vi "color split.vi"(4 "point style":enum16{"dot", "cross"}(ring), 5 "mapping":T1(ring), 6 "tfolder":T3={"tfolder path"=path "/snowfall/Users/arcadi/Desktop/Ultrasound/Experiment/YBCO_4/Round1/Sweep12/June_2011/062511/221.16400K_300_3100_001_062511.dat", "9folder path"=path "/snowfall/Users/arcadi/Desktop/Ultrasound/Experiment/YBCO_4/Round1/Sweep12/June_2011/062511/221.16400K_300_3100_001_062511.dat", "tfolder  -  file array"=[], "from index array"=[], "timestamp array"=[]}, 7 "Plot Ref":refnum<vi>, 8 "plot array IN":T2(array[cluster]), 10 "Y":dbl[](array[numeric]), 11 "X":dbl[](array[numeric])) -> (0 "plot array OUT":T2(array[cluster]))   [LabVIEW 2015]
uses:
  tfolder.ctl
  tfolder -- monotonic segment.ctl
panel:
  in  "output cluster":T5
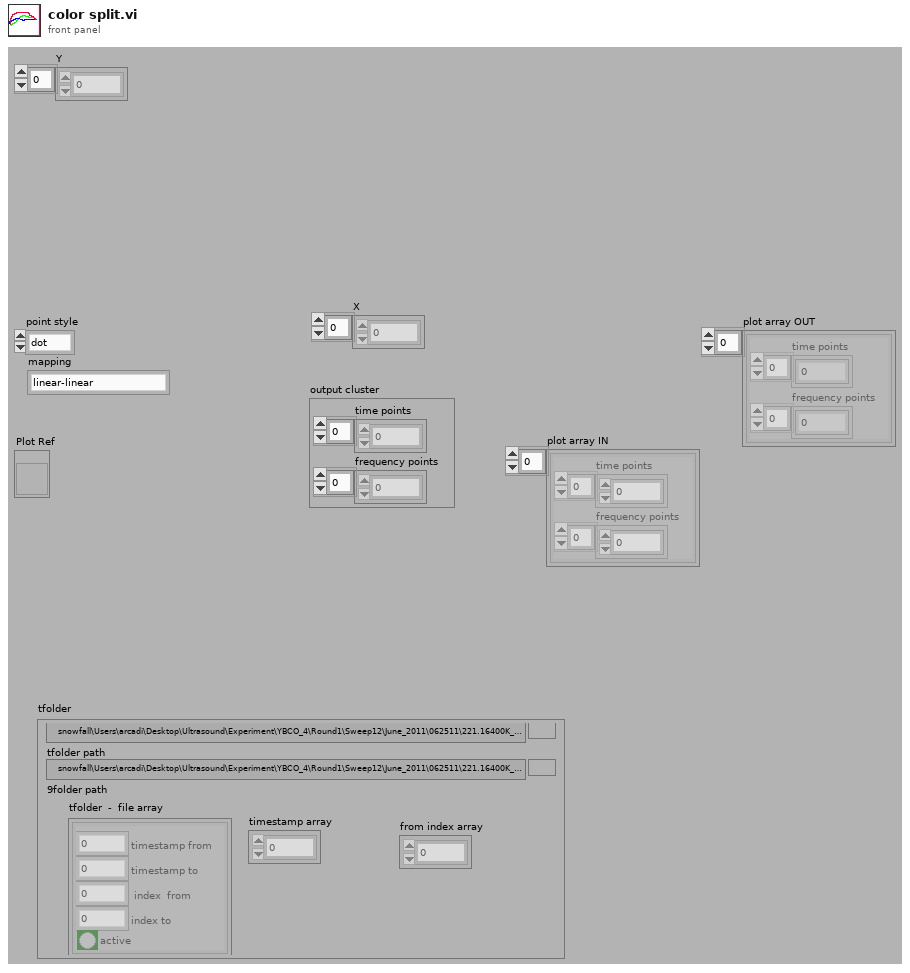
[diagram p1: front panel]
types:
  T1 = enum16{"linear-linear", "log-linear", "linear-log", "log-log"}
  T2 = cluster{"time points":dbl[], "frequency points":dbl[]}[]
  T3 = typedef "tfolder.ctl" = cluster{"tfolder path":path, "9folder path":path, "tfolder  -  file array":T4[], "from index array":i32[], "timestamp array":dbl[]}
  T4 = typedef "tfolder -- monotonic segment.ctl" = cluster{"timestamp from":dbl, "timestamp to":dbl, " index  from":i32, "index to":i32, "active":bool}
  T5 = cluster{"time points":dbl[], "frequency points":dbl[]}
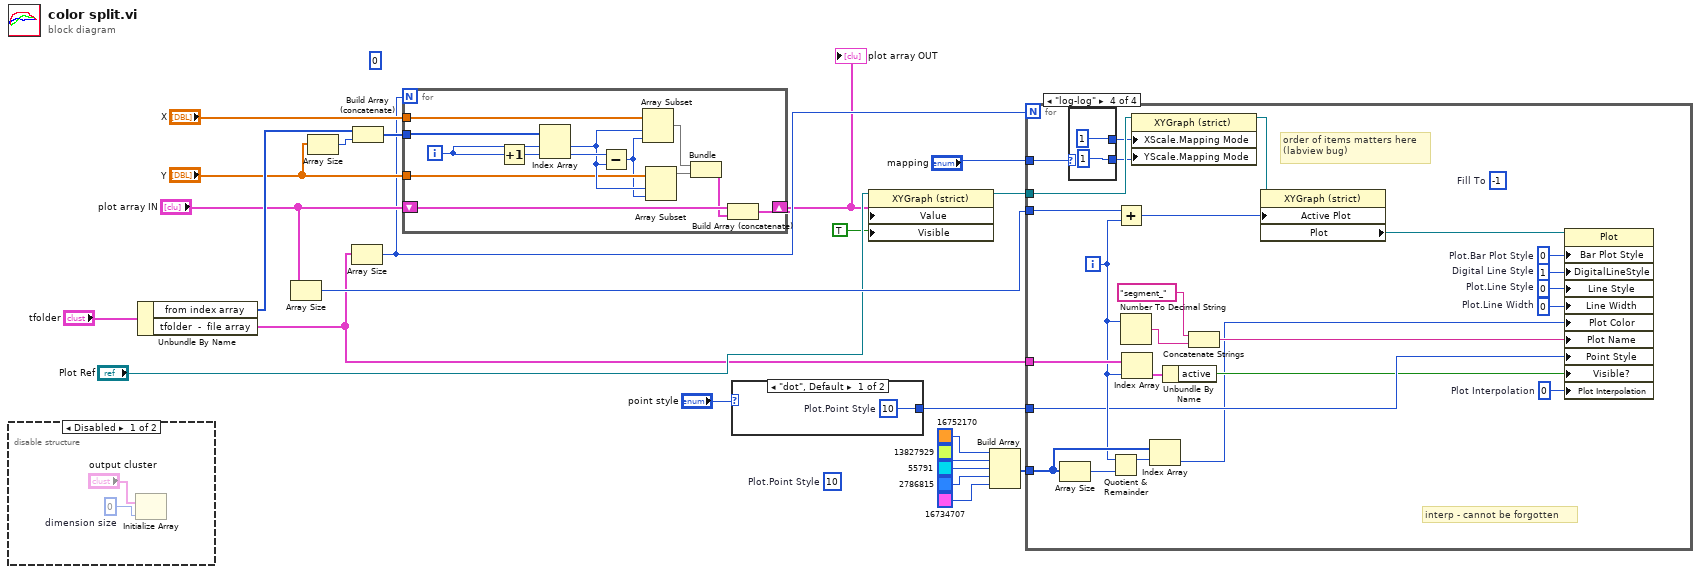
[diagram p0: block diagram]
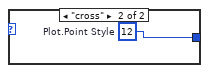
[diagram p2: hidden frame]
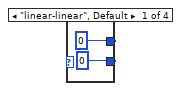
[diagram p4: hidden frame]
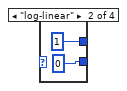
[diagram p5: hidden frame]
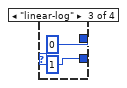
[diagram p6: hidden frame]
diagram:
  (unwired) u8 10  # Plot.Point Style
  (unwired) 0 ("dimension size")
  n1 = disable-structure shown="Disabled" {
    frame Disabled {
      w25 = 0  # dimension size
      n2 = Initialize Array("output cluster", w25) -> ()  [unwired: 1 out]
    }
    frame Enabled {
    }
  }
  n3 = Unbundle By Name("tfolder") -> ("from index array"=w21:i32[], "tfolder  -  file array"=w6:T4[])
  n4 = Array Size(array="plot array IN") -> (size(s)=w16:i32)
  n5 = Array Size(array="Y") -> (size(s)=w22:i32)
  n6 = Array Size(array=w6) -> (size(s)=w9:i32)
  n7 = Build Array (concatenate)(w21, w22) -> (w20:i32[])
  n8 = for {
    N: w9 -> [_]
    shift-right: [w31] -> w7
    shift-left: "plot array IN" -> [w32]
    tunnel: w20 -> [w38]
    tunnel: "X" -> [w36]
    tunnel: "Y" -> [w33]
    i -> [w26]
    n9 = Increment(x=w26) -> (x+1=w37:i32)
    n10 = Index Array(array=w38, index #1=w26, index #2=w37) -> (element #1=w34:i32, element #2=w35:i32)
    n11 = Subtract(x=w35, y=w34) -> (x-y=w29:i32)
    n12 = Array Subset(array=w36, index=w34, length=w29) -> (w30:dbl[])
    n13 = Array Subset(array=w33, index=w34, length=w29) -> (w28:dbl[])
    n14 = Bundle(w30, w28) -> (w27:cluster{dbl[], dbl[]})  [unwired: 1 in]
    n15 = Build Array (concatenate)(w32, w27) -> (w31:T2)
  }
  "plot array OUT" <- w7
  n16 = case shown="\"dot\", Default" "point style" {
    tunnel: [w39 w40] -> w3
    frame "dot", Default {
      w39 = u8 10  # Plot.Point Style
    }
    frame "cross" {
      w40 = u8 12  # Plot.Point Style
    }
  }
  n17 = property on="Property Node" class="XYGraph (strict)"(reference="Plot Ref", "Value"=w7, "Visible"=TRUE) -> (reference out=w5:refnum<vi>)  [unwired: 1 in, 1 out]
  n18 = Build Array(u32 16752170, u32 13827929, u32 55791, u32 2786815, u32 16734707) -> (w10:u32[])
  n19 = for {
    N: w9 -> [_]
    tunnel: w6 -> [w59]
    tunnel: w16 -> [w61]
    tunnel: w10 -> [w60]
    tunnel: w5 -> [w44]
    tunnel: w3 -> [w55]
    tunnel: "mapping" -> [w45]
    i -> [w56]
    w46 = u8 0  # Plot Interpolation
    (unwired) i16 -1  # Fill To
    w54 = u8 1  # Digital Line Style
    w52 = u8 0  # Plot.Line Width
    w51 = u8 0  # Plot.Line Style
    w50 = u8 0  # Plot.Bar Plot Style
    # "interp - cannot be forgotten"
    # "order of items matters here \n(labview bug)"
    n20 = Array Size(array=w60) -> (size(s)=w63:i32)
    n21 = case shown="\"log-log\"" w45 {
      tunnel: [u8 0 ("X Scale.Mapping Mode") u8 1 ("X Scale.Mapping Mode") u8 0 ("X Scale.Mapping Mode") u8 1 ("X Scale.Mapping Mode")] -> w42
      tunnel: [u8 0 ("X Scale.Mapping Mode") u8 0 ("X Scale.Mapping Mode") u8 1 ("X Scale.Mapping Mode") u8 1 ("X Scale.Mapping Mode")] -> w41
      frame "linear-linear", Default {
      }
      frame "log-linear" {
      }
      frame "linear-log" {
      }
      frame "log-log" {
      }
    }
    n22 = Quotient & Remainder(x=w56, y=w63) -> (x-y*floor(x/y)=w62:i32)  [unwired: 1 out]
    n23 = Add(x=w61, y=w56) -> (x+y=w64:i32)
    n24 = Number To Decimal String(number=w56) -> (decimal integer string=w58:string)  [unwired: 1 in]
    n25 = Index Array(array=w59, index=w56) -> (element=w65:T4)
    n26 = property on="Property Node" class="XYGraph (strict)"(reference=w44, "XScale.Mapping Mode"=w42, "YScale.Mapping Mode"=w41) -> (reference out=w43:refnum<vi>)  [unwired: 1 in, 1 out]
    n27 = Index Array(array=w60, index=w62) -> (element=w48:u32)
    n28 = Unbundle By Name(w65) -> ("active"=w53:bool)
    n29 = Concatenate Strings("segment_", w58) -> (w49:string)
    n30 = property on="Property Node" class="XYGraph (strict)"(reference=w43, "Active Plot"=w64) -> ("Plot"=w47:refnum<vi>)  [unwired: 1 in, 2 out]
    n31 = property class="Plot"(reference=w47, "Bar Plot Style"=w50, "DigitalLineStyle"=w54, "Line Style"=w51, "Line Width"=w52, "Plot Color"=w48, "Plot Name"=w49, "Point Style"=w55, "Visible?"=w53, "Plot Interpolation"=w46) -> ()  [unwired: 1 in, 2 out]
  }
